vi "Run Bfr Rx - Untimed.vi"(7 "Process in":refnum<class "Process.lvclass">, 8 "error in (no error)":errorcluster, 11 "Rx Loop Data in":T1 {"Buffer Resources"."Data Buffer" format="%016x"; "Buffer Option Support"."Ping Pong Buffer"."Buffer_B" format="%016x"; "Buffer Option Support"."Cached Buffer"."Cache Buffer" format="%016x"}) -> (3 "Rx Loop Data out":T1 {"Buffer Resources"."Data Buffer" format="%016x"; "Buffer Option Support"."Ping Pong Buffer"."Buffer_B" format="%016x"; "Buffer Option Support"."Cached Buffer"."Cache Buffer" format="%016x"})   [LabVIEW 2016, in "UDP-Custom-Device Engine.lvlib"]
uses:
  UDP-Custom-Device Engine.lvlib
  <vilib>/NI/NIVS Inline Async API/_VS Inline Async API/Process/Process.lvclass
  Types/Engine - Buffered Rx Loop Data.ctl
  Types/Engine - General Resources.ctl
  <vilib>/NI Veristand/VeriStand Data/Typedefs/Typedefs.Data Types.ctl
  Shared/Types/Shared - Duplex Settings.ctl
  Shared/Types/Shared - Header Details.ctl
  Types/Engine - Buffer Resources.ctl
  Shared/Types/Shared - Pointer Encoding.ctl
  Types/Engine - Rx Runtime Resources.ctl
  Types/Engine - Execution Config.ctl
  Shared/Types/Shared - Thread Management.ctl
  Types/Engine - Rx New Data Options Support.ctl
  Shared/Types/Shared - New Data Options.ctl
  Types/Engine - Buffered Rx Buffer Option Support.ctl
  Shared/Types/Shared - Receive Buffer Options.ctl
  Types/Engine - Buffered Rx Circular Buffer.ctl
  Types/Engine - Buffered Rx Cached Buffer.ctl
  Types/Engine - Buffered Rx Ping Pong Buffer.ctl
  Types/Engine - Buffered Rx Active Buffer.ctl
  <vilib>/NI/NIVS Inline Async API/_Data Access Engine/Data Access Engine/Types/Read.DVR.ctl
  <vilib>/NI/NIVS Inline Async API/_Data Access Engine/Access Type Classes/Read/Read.lvclass
  <vilib>/NI/NIVS Inline Async API/_Data Access Engine/Data Access Engine/Types/Write.DVR.ctl
  <vilib>/NI/NIVS Inline Async API/_Data Access Engine/Access Type Classes/Write/Write.lvclass
  Types/Engine - Buffered Rx Channel Refs.ctl
  Types/Engine - Debug Resources.ctl
  <vilib>/NI/NIVS Inline Async API/_Data Access Engine/Access Type Classes/Read/Read.lvclass/Read.ctl
  <vilib>/NI/NIVS Inline Async API/_Data Access Engine/Access Type Classes/Write/Write.lvclass/Write.ctl
  <vilib>/NI/NIVS Inline Async API/_VS Inline Async API/Process/Process.lvclass/Process.ctl
  <vilib>/NI Veristand/VeriStand Data/Type Conversion/Type Conversion.To Double (U64).vi
  <vilib>/NI/NIVS Inline Async API/_Data Access Engine/Data Access Engine/Methods/Write.Data.vi
  <vilib>/NI/NIVS Inline Async API/_Data Access Engine/Data Access Engine/Methods/Read.Data.vi
  <vilib>/NI Veristand/VeriStand Data/Pointer Operations/Pointer.Write.vi
  <vilib>/NI Veristand/VeriStand Data/Pointer Operations/Pointer.Write (1D U8).vi
  Run Bfr Rx - Handle Offset.vi
  Run Bfr Rx - Handle Rollover.vi
  Circular Buffer and Size/Run Bfr Rx - Sized Detect Rollover.vi
  Circular Buffer and Size/Run Bfr Rx - Sized Handle Rollover.vi
  Circular Buffer and Size/Run Bfr Rx - Sized Write Buffer.vi
  Block Cache and Size/Run Bfr Rx - Cached - Check Cache.vi
  Block Cache and Size/Run Bfr Rx - Cached - Copy Flush Add.vi
  Block Cache and Size/Run Bfr Rx - CachedSize - Check Cache.vi
  Block Cache and Size/Run Bfr Rx - CachedSize - Copy Flush Add.vi
  <vilib>/NI/NIVS Inline Async API/_Data Access Engine/Access Type Classes/Write/Write.ProcessData.vi
  <vilib>/NI Veristand/VeriStand Data/Type Conversion/Type Conversion.To Double (U16).vi
  <vilib>/NI/NIVS Inline Async API/_VS Inline Async API/Error Handling Process/SubVIs/Error.ConvertArray.vi
  <vilib>/NI/NIVS Inline Async API/_Data Access Engine/Access Type Classes/Read/Read.ProcessData.vi
  <vilib>/NI Veristand/VeriStand Data/Pointer Operations/Pointer.Write (I32).vi
  Block Cache and Size/Run Bfr Rx - Cached - Copy Cache.vi
  Block Cache and Size/Run Bfr Rx - Cached - Flush Cache.vi
  Block Cache and Size/Run Bfr Rx - Cached - Add to Cache.vi
  Block Cache and Size/Run Bfr Rx - CachedSize - Copy Cache.vi
  Block Cache and Size/Run Bfr Rx - CachedSize - Flush Cache.vi
  Block Cache and Size/Run Bfr Rx - CachedSize - Add to Cache.vi
  <vilib>/NI Veristand/VeriStand Data/Pointer Operations/Pointer.In-Place Read.vi
  <vilib>/NI Veristand/VeriStand Data/Pointer Operations/Pointer.In-Place Read (1D U8).vi
  <vilib>/NI Veristand/VeriStand Data/Pointer Operations/Pointer.Read.vi
  <vilib>/NI Veristand/VeriStand Data/Pointer Operations/Pointer.Read (U16).vi
  <vilib>/NI Veristand/VeriStand Data/Pointer Operations/Pointer.Write (U16).vi
  <vilib>/NI Veristand/VeriStand Data/Pointer Operations/Pointer.In-Place Read (U16).vi
  <vilib>/NI Veristand/VeriStand Data/VeriStand Data.lvlib
  <vilib>/NI/NIVS Inline Async API/_Data Access Engine/Data Access Engine/Data Access Engine.lvclass
  Shared/UDP-Custom-Device Shared.lvlib
panel:
  out "dataBuffer":u64 format="%016x"
  out "dataLength":u64
  out "Tx Packet":string
  # "BUFFERED RECEIVE\n- UNTIMED\n- ALL TARGETS"
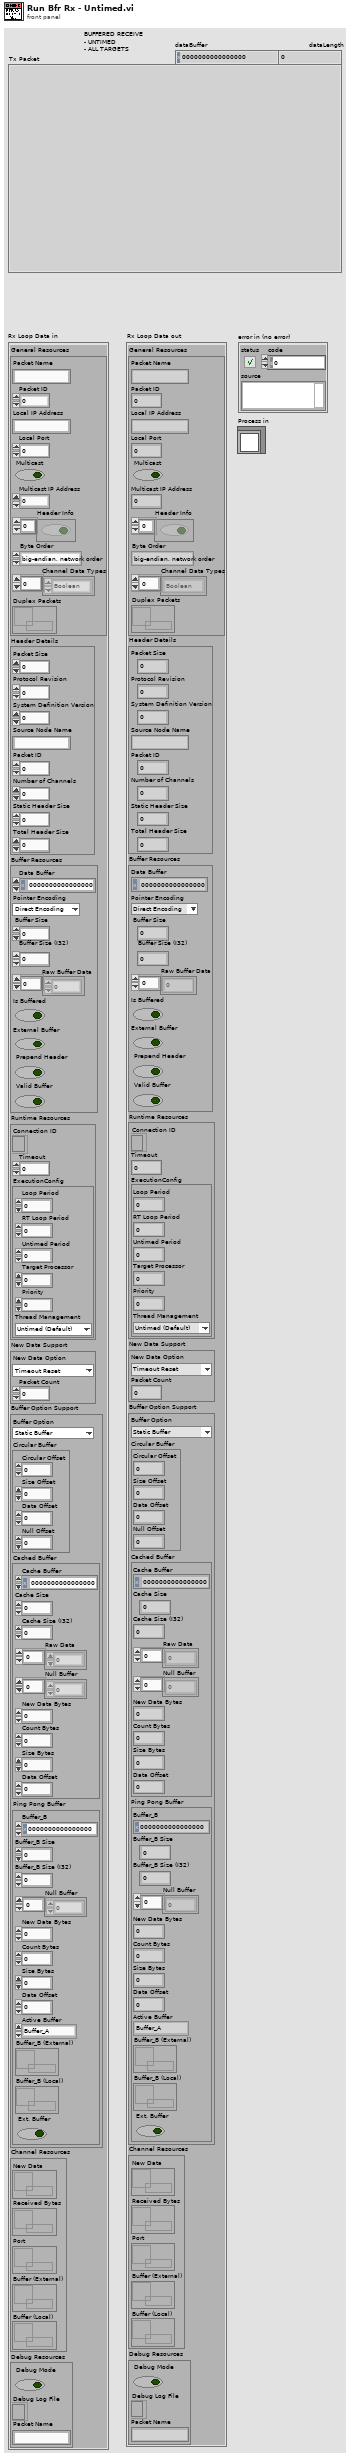
[diagram p1: front panel]
types:
  T1 = typedef "UDP-Custom-Device Engine.lvlib/Engine - Buffered Rx Loop Data.ctl" = cluster{"General Resources":T2, "Header Details":T4, "Buffer Resources":T5, "Runtime Resources":T7, "New Data Support":T10, "Buffer Option Support":T12, "Channel Resources":T20, "Debug Resources":T21}
  T2 = typedef "UDP-Custom-Device Engine.lvlib/Engine - General Resources.ctl" = cluster{"Packet Name":string, "Packet ID":i32, "Local IP Address":string, "Local Port":i32, "Multicast":bool, "Multicast IP Address":u32, "Header Info":bool[], "Byte Order":enum16{"big-endian, network order", "native, host order", "little-endian"}, "Channel Data Types":T3[], "Duplex Packets":refnum<data-value>}
  T3 = typedef "VeriStand Data.lvlib/Typedefs.Data Types.ctl" = enum16{"Boolean", "Single", "Double", "I8", "I16", "I32", "I64", "U8", "U16", "U32", "U64"}
  T4 = typedef "UDP-Custom-Device Shared.lvlib/Shared - Header Details.ctl" = cluster{"Packet Size":u16, "Protocol Revision":u8, "System Definition Version":u64, "Source Node Name":string, "Packet ID":u32, "Number of Channels":u32, "Static Header Size":u16, "Total Header Size":u16}
  T5 = typedef "UDP-Custom-Device Engine.lvlib/Engine - Buffer Resources.ctl" = cluster{"Data Buffer":u64, "Pointer Encoding":T6, "Buffer Size":u64, "Buffer Size (I32)":i32, "Raw Buffer Data":u8[], "Is Buffered":bool, "External Buffer":bool, "Prepend Header":bool, "Valid Buffer":bool}
  T6 = typedef "UDP-Custom-Device Shared.lvlib/Shared - Pointer Encoding.ctl" = enum16{"Direct Encoding", "Conversion Encoding"}
  T7 = typedef "UDP-Custom-Device Engine.lvlib/Engine - Rx Runtime Resources.ctl" = cluster{"Connection ID":refnum<k16>, "Timeout":i32, "ExecutionConfig":T8}
  T8 = typedef "UDP-Custom-Device Engine.lvlib/Engine - Execution Config.ctl" = cluster{"Loop Period":i64, "RT Loop Period":i64, "Untimed Period":u32, "Target Processor":i32, "Priority":i32, "Thread Management":T9}
  T9 = typedef "UDP-Custom-Device Shared.lvlib/Shared - Thread Management.ctl" = enum16{"Untimed (Default)", "Timed (High Priority)"}
  T10 = typedef "UDP-Custom-Device Engine.lvlib/Engine - Rx New Data Options Support.ctl" = cluster{"New Data Option":T11, "Packet Count":dbl}
  T11 = typedef "UDP-Custom-Device Shared.lvlib/Shared - New Data Options.ctl" = enum16{"Timeout Reset", "Counter"}
  T12 = typedef "UDP-Custom-Device Engine.lvlib/Engine - Buffered Rx Buffer Option Support.ctl" = cluster{"Buffer Option":T13, "Circular Buffer":T14, "Cached Buffer":T15, "Ping Pong Buffer":T16}
  T13 = typedef "UDP-Custom-Device Shared.lvlib/Shared - Receive Buffer Options.ctl" = enum16{"Static Buffer", "Circular Buffer", "Circular Buffer + Size", "Internal Cache", "Internal Cache + Size", "Ping Pong", "Ping Pong + Size"}
  T14 = typedef "UDP-Custom-Device Engine.lvlib/Engine - Buffered Rx Circular Buffer.ctl" = cluster{"Circular Offset":u64, "Size Offset":u64, "Data Offset":u64, "Null Offset":u64}
  T15 = typedef "UDP-Custom-Device Engine.lvlib/Engine - Buffered Rx Cached Buffer.ctl" = cluster{"Cache Buffer":u64, "Cache Size":u64, "Cache Size (I32)":i32, "Raw Data":u8[], "Null Buffer":u8[], "New Data Bytes":u64, "Count Bytes":u64, "Size Bytes":u64, "Data Offset":u64}
  T16 = typedef "UDP-Custom-Device Engine.lvlib/Engine - Buffered Rx Ping Pong Buffer.ctl" = cluster{"Buffer_B":u64, "Buffer_B Size":u64, "Buffer_B Size (I32)":i32, "Null Buffer":u8[], "New Data Bytes":u64, "Count Bytes":u64, "Size Bytes":u64, "Data Offset":u64, "Active Buffer":T17, "Buffer_B (External)":T18, "Buffer_B (Local)":T19, "Ext. Buffer":bool}
  T17 = typedef "UDP-Custom-Device Engine.lvlib/Engine - Buffered Rx Active Buffer.ctl" = enum16{"Buffer_A", "Buffer_B"}
  T18 = typedef "Data Access Engine.lvlib/Data Access Engine.lvclass/Read.DVR.ctl" = refnum<data-value>
  T19 = typedef "Data Access Engine.lvlib/Data Access Engine.lvclass/Write.DVR.ctl" = refnum<data-value>
  T20 = typedef "UDP-Custom-Device Engine.lvlib/Engine - Buffered Rx Channel Refs.ctl" = cluster{"New Data":T19, "Received Bytes":T19, "Port":T19, "Buffer (External)":T18, "Buffer (Local)":T19}
  T21 = typedef "UDP-Custom-Device Engine.lvlib/Engine - Debug Resources.ctl" = cluster{"Debug Mode":bool, "Debug Log File":refnum<file>, "Packet Name":string}
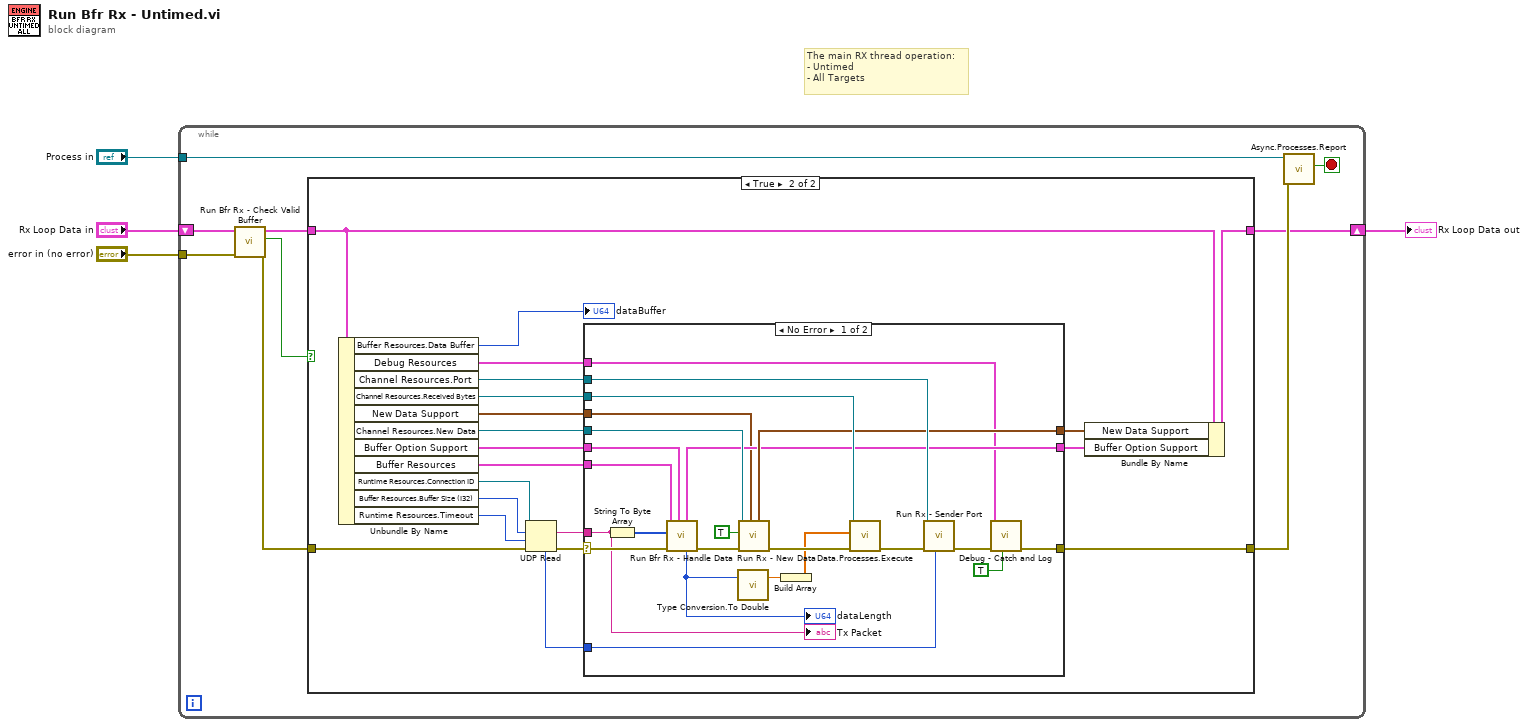
[diagram p0: block diagram]
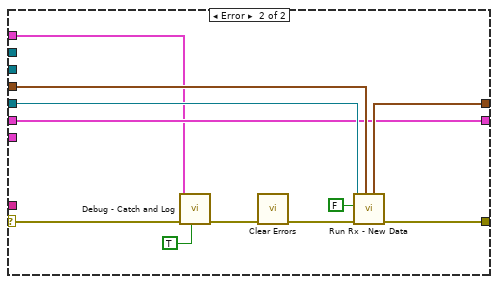
[diagram p3: hidden frame]
diagram:
  # "The main RX thread operation:\n- Untimed\n- All Targets"
  n1 = while {
    tunnel: "error in (no error)" -> [w6]
    tunnel: "Process in" -> [w13]
    shift-right: [w10] -> w3
    shift-left: "Rx Loop Data in" -> [w9]
    stop <- w12 stop-if-true
    n2 = call "Run Bfr Rx - Check Valid Buffer.vi"("error in (no error)"=w6, "Rx Loop Data in"=w9) -> ("error out"=w5:errorcluster, "Allow Rx?"=w7:bool, "Rx Loop Data out"=w8:T1)  [unwired: 7 in]
    n3 = case shown="True" w7 {
      tunnel: w8 -> [w14 w25]
      tunnel: w5 -> [w15 w33]
      tunnel: [w15 w31] -> w11
      tunnel: [w14 w24] -> w10
      frame False {
        # "Invalid buffer. Wait for us to have one that we can use."
      }
      frame True {
        n4 = Unbundle By Name(w25) -> ("Buffer Resources.Data Buffer"=→"dataBuffer":u64, "Debug Resources"=w21:T21, "Channel Resources.Port"=w27:T19, "Channel Resources.Received Bytes"=w28:T19, "New Data Support"=w20:T10, "Channel Resources.New Data"=w29:T19, "Buffer Option Support"=w22:T12, "Buffer Resources"=w19:T5, "Runtime Resources.Connection ID"=w35:refnum<k16>, "Buffer Resources.Buffer Size (I32)"=w17:i32, "Runtime Resources.Timeout"=w34:i32)
        n5 = UDP Read(connection ID=w35, max size (548)=w17, timeout ms (25000)=w34, 8:w33) -> (data out=w32:string, error out=w30:errorcluster, 4:w26:u16)  [unwired: 2 out]
        n6 = case shown="No Error" w30 {
          selector: w30 -> [w47 w61]
          tunnel: w22 -> [w44 w63]
          tunnel: w32 -> [w36 _]
          tunnel: [w40 w66] -> w31
          tunnel: w29 -> [w58 w68]
          tunnel: w28 -> [w56 _]
          tunnel: w27 -> [w52 _]
          tunnel: w26 -> [w50 _]
          tunnel: w20 -> [w39 w65]
          tunnel: [w49 w64] -> w23
          tunnel: [w45 w63] -> w18
          tunnel: w21 -> [w42 w59]
          tunnel: w19 -> [w38 _]
          frame No Error {
            n7 = String To Byte Array(string=w36) -> (unsigned byte array=w48:u8[])
            n8 = call "Run Bfr Rx - Handle Data.vi"("Buffer Option Support in"=w44, "error in (no error)"=w47, "Data"=w48, "Buffer Resources"=w38) -> ("error out"=w46:errorcluster, "Data Size"=w37:u64, "Buffer Option Support out"=w45:T12)  [unwired: 5 in]
            "dataLength" <- w37
            n9 = call-poly <vilib>:"Type Conversion.To Double.vi"("value in"=w37) -> ("value out"=w54:dbl)  [unwired: 2 in]
            n10 = call "Run Rx - New Data.vi"("New Data Support in"=w39, "error in (no error)"=w46, "New Data"=TRUE, "New Data Ref"=w58) -> ("error out"=w55:errorcluster, "New Data Support out"=w49:T10)  [unwired: 6 in]
            n11 = Build Array(w54) -> (w53:dbl[])
            n12 = call-poly <vilib>:"Data.Processes.Execute.vi"("error in (no error)"=w55, "Values"=w53, "Ref"=w56) -> ("error out"=w51:errorcluster)  [unwired: 8 in]
            n13 = call "Run Rx - Sender Port.vi"("Port"=w50, "error in (no error)"=w51, "Port Ref"=w52) -> ("error out"=w41:errorcluster)  [unwired: 8 in]
            n14 = call "Debug - Catch and Log.vi"("Clear Error?"=TRUE, "error in (no error)"=w41, "Debug Resources"=w42) -> ("error out"=w40:errorcluster)  [unwired: 8 in]
            "Tx Packet" <- w36
          }
          frame Error {
            n15 = call "Debug - Catch and Log.vi"("Clear Error?"=TRUE, "error in (no error)"=w61, "Debug Resources"=w59) -> ("error out"=w60:errorcluster)  [unwired: 8 in]
            n16 = call <vilib>:"Clear Errors.vi"("error in (no error)"=w60) -> ("error out"=w67:errorcluster)  [unwired: 5 in, 1 out]
            n17 = call "Run Rx - New Data.vi"("New Data Support in"=w65, "error in (no error)"=w67, "New Data"=FALSE, "New Data Ref"=w68) -> ("error out"=w66:errorcluster, "New Data Support out"=w64:T10)  [unwired: 6 in]
          }
        }
        n18 = Bundle By Name(cluster=w25, "New Data Support"=w23, "Buffer Option Support"=w18) -> (w24:T1)
      }
    }
    n19 = call <vilib>:"Async.Processes.Report.vi"("Error"=w11, "Process in"=w13) -> ("Stop"=w12:bool)  [unwired: 8 in, 1 out]
  }
  "Rx Loop Data out" <- w3
